vi "Cam Ini (SubVI).vi"(8 "error in":errorcluster, 10 "VideoMode":u32, 11 "Camera":T2) -> (0 "error out":errorcluster, 2 "Image Ref":T1, 3 "Cam Ref":T2)   [LabVIEW 2013]
uses:
  <vilib>/userdefined/High Color/IMAQdx.ctl
  <vilib>/vision/Image Controls.llb/IMAQ Image.ctl
  <vilib>/vision/driver/IMAQdx.llb/IMAQdx Acquisition Mode.ctl
  <vilib>/vision/driver/NI_Vision_Acquisition_Software.lvlib
  <resource>/objmgr/imaqdx.rc
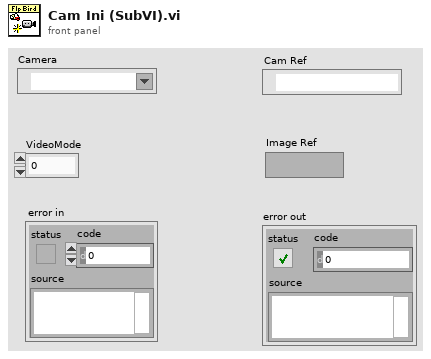
[diagram p1: front panel]
types:
  T1 = typedef "IMAQ Image.ctl" = refnum<image>
  T2 = typedef "IMAQdx.ctl" = refnum<k21>
  T3 = typedef "Image Type" = u32
  T4 = typedef "NI_Vision_Acquisition_Software.lvlib/IMAQdx Acquisition Mode.ctl" = enum32{"One Shot", "Continuous"}
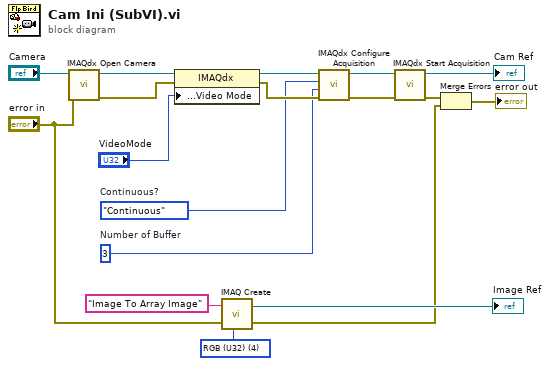
[diagram p0: block diagram]
diagram:
  w5 = T3 4 items=["Grayscale (U8)", "Grayscale (I16)", "Grayscale (SGL)", "Complex (CSG)", "RGB (U32)", "HSL (U32)", "RGB (U64)", "Grayscale (U16)"] ("Image Type")
  w11 = IMAQdx_Acquisition_Mode."Continuous"  # Continuous?
  w8 = u32 3  # Number of Buffer
  n1 = call <vilib>:"IMAQdx Open Camera.vi"("error in"="error in", "Session In"="Camera") -> ("error out"=w17:errorcluster, "Session Out"=w15:T2)  [unwired: 1 in, 7 out]
  n2 = property class="IMAQdx"(reference=w15, error in=w17, "Acquisition Attributes:Video Mode"="VideoMode") -> (reference out=w16:T2, error out=w18:errorcluster)
  n3 = call "IMAQ Create"("Image Name"="Image To Array Image", "Image Type"=w5, "error in (no error)"="error in") -> ("New Image"=→"Image Ref":T1, "error out"=w1:errorcluster)  [unwired: 2 in]
  n4 = call <vilib>:"IMAQdx Configure Acquisition.vi"("error in"=w18, "Number of Buffers"=w8, "Continuous?"=w11, "Session In"=w16) -> ("error out"=w14:errorcluster, "Session Out"=w13:T2)  [unwired: 6 out]
  n5 = call <vilib>:"IMAQdx Start Acquisition.vi"("error in"=w14, "Session In"=w13) -> ("error out"=w9:errorcluster, "Session Out"=→"Cam Ref":T2)  [unwired: 8 out]
  n6 = Merge Errors(w9, w1) -> (→"error out":errorcluster)
